vi "Clear Graph.vi"(8 "error in (no error)":errorcluster, 11 "Graph Manager in":refnum<class "Graph Manager.lvclass">) -> (0 "error out":errorcluster, 3 "Graph Manager out":refnum<class "Graph Manager.lvclass">)   [LabVIEW 2016, in "Graph Manager.lvclass"]
uses:
  Graph Manager.lvclass
  Graph Manager.lvclass/Graph Manager.ctl
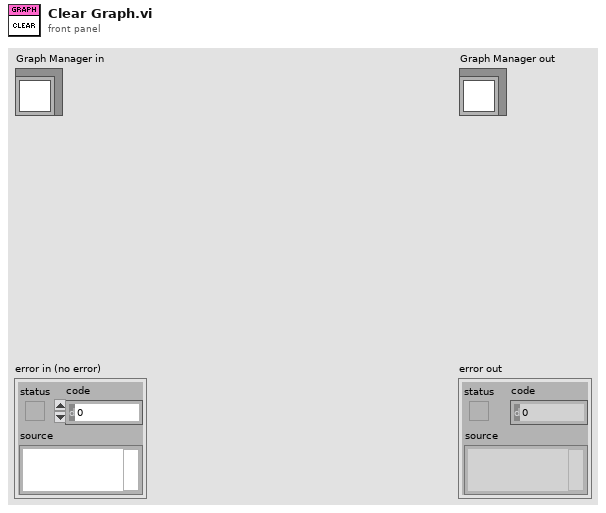
[diagram p1: front panel]
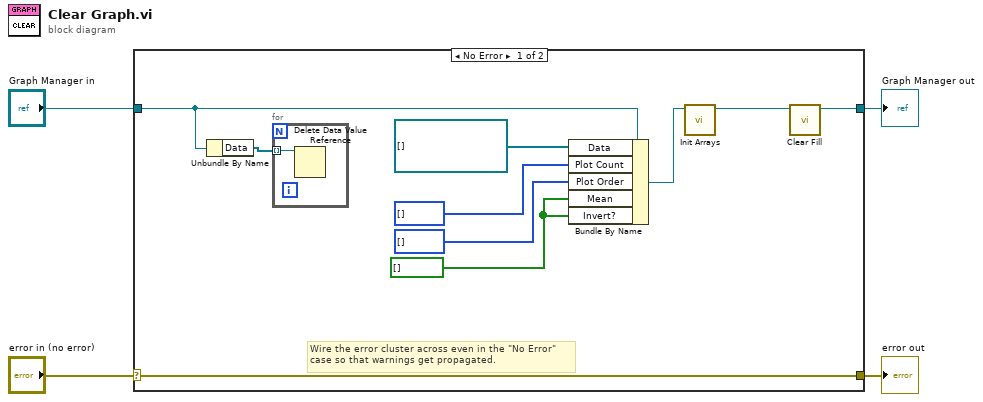
[diagram p0: block diagram]
diagram:
  n1 = case shown="No Error" "error in (no error)" {
    selector: "error in (no error)" -> [w14 w17]
    tunnel: [w14 w17] -> w3
    tunnel: [w6 w16] -> w1
    tunnel: "Graph Manager in" -> [w12 w16]
    frame No Error {
      w5 = bool[] [] ("Mean")
      # "Wire the error cluster across even in the \"No Error\"\ncase so that warnings get propagated."
      n2 = Unbundle By Name(w12) -> ("Data"=w13:refnum<data-value>[])
      n3 = for {
        tunnel: w13 -> [w15] mode=indexing
        n4 = Delete Data Value Reference(data value reference=w15) -> ()  [unwired: 1 in, 2 out]
      }
      n5 = Bundle By Name(cluster=w12, "Data"=refnum<data-value>[] [], "Plot Count"=i32[] [], "Plot Order"=i32[] [], "Mean"=w5, "Invert?"=w5) -> (w8:refnum<class "Graph Manager.lvclass">)
      n6 = call-dynamic "Init Arrays.vi"("Graph Manager in"=w8) -> ("Graph Manager out"=w7:refnum<class "Graph Manager.lvclass">)  [unwired: 9 in, 1 out]
      n7 = call "Clear Fill.vi"("Graph Manager in"=w7) -> ("Graph Manager out"=w6:refnum<class "Graph Manager.lvclass">)  [unwired: 9 in, 1 out]
    }
    frame Error {
    }
  }
  "error out" <- w3
  "Graph Manager out" <- w1
